vi "EditorThumbnail deleteElement.vi"(8 "error in (no error)":errorcluster, 11 "EditorThumbnail in":refnum<class "EditorThumbnail.lvclass">) -> (0 "error out":errorcluster, 3 "EditorThumbnail out":refnum<class "EditorThumbnail.lvclass">)   [LabVIEW 2018, in "EditorThumbnail.lvclass"]
uses:
  EditorThumbnail.lvclass
  EditorThumbnail.lvclass/EditorThumbnail.ctl
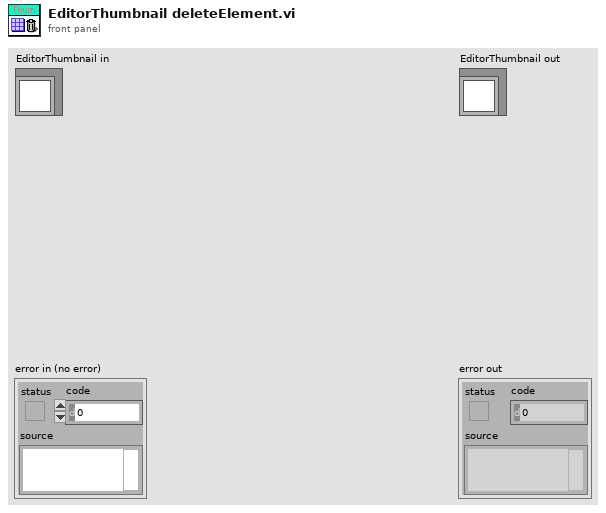
[diagram p1: front panel]
types:
  T1 = cluster{"index":u32, "data":cluster{"xdata":dbl[], "ydata":sgl[]}[], "peak":dbl[], "picture":picture}[]
  T2 = cluster{"index":u32, "data":cluster{"xdata":dbl[], "ydata":sgl[]}[], "peak":dbl[], "picture":picture}
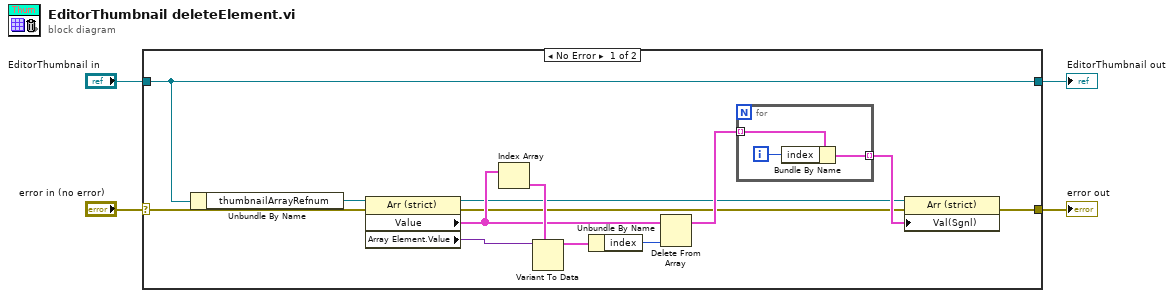
[diagram p0: block diagram]
diagram:
  n1 = case shown="No Error" "error in (no error)" {
    selector: "error in (no error)" -> [w13 w22]
    tunnel: [w15 w22] -> w3
    tunnel: [w17 w21] -> w1
    tunnel: "EditorThumbnail in" -> [w17 w21]
    frame No Error {
      n2 = Unbundle By Name(w17) -> ("thumbnailArrayRefnum"=w14:refnum<vi>)
      n3 = property class="Arr (strict)"(reference=w14, error in=w13) -> (reference out=w6:refnum<vi>, error out=w5:errorcluster, "Value"=w10:T1, "Array Element.Value"=w11:variant)
      n4 = Index Array(array=w10) -> (element=w12:T2)  [unwired: 1 in]
      n5 = Variant To Data(type=w12, Variant=w11) -> (data=w9:T2)  [unwired: 1 in, 1 out]
      n6 = Unbundle By Name(w9) -> ("index"=w8:u32)
      n7 = Delete From Array(array=w10, index=w8) -> (array with subset deleted=w7:T1)  [unwired: 1 in, 1 out]
      n8 = for {
        tunnel: w7 -> [w18] mode=indexing
        tunnel: [w20] -> w16 mode=indexing
        i -> [w19]
        n9 = Bundle By Name(cluster=w18, "index"=w19) -> (w20:T2)
      }
      n10 = property class="Arr (strict)"(reference=w6, error in=w5, "Val(Sgnl)"=w16) -> (error out=w15:errorcluster)  [unwired: 1 out]
    }
    frame Error {
    }
  }
  "error out" <- w3
  "EditorThumbnail out" <- w1
